vi "Read Plot reference.vi"(9 "Plot in":refnum<class "Plot.lvclass">) -> (3 "Plot out":refnum<class "Plot.lvclass">, 4 "Plot reference":refnum<vi>)   [LabVIEW 2014, in "Raspberry Pi Compatible Compiler for LabVIEW.lvlib" / "Plot.lvclass"]
uses:
  Plot.lvclass
  Plot.lvclass/Plot.ctl
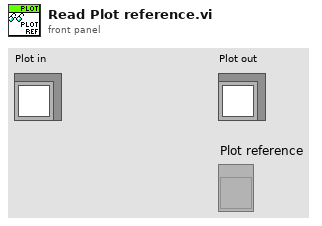
[diagram p1: front panel]
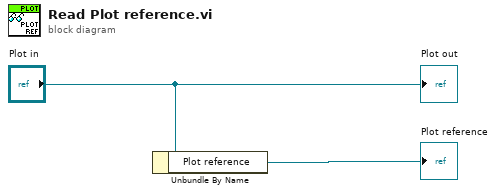
[diagram p0: block diagram]
diagram:
  n1 = Unbundle By Name("Plot in") -> ("Plot reference"=→"Plot reference":refnum<vi>)
  "Plot out" <- "Plot in"
